vi "stop_pico_acq.vi"() -> ()   [LabVIEW 2015]
panel:
  in  "stop_pico_acq":bool
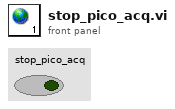
[diagram p1: front panel]
diagram:
